vi "DB - T-SQL Query.vi"(8 "error in (no error)":errorcluster, 10 "T-SQL":string, 11 "connection reference":T1) -> (0 "error out":errorcluster, 2 "2D data":string[][](array[string]), 3 "connection reference":T1)   [LabVIEW 2020]
uses:
  <vilib>/addons/database/Connection.llb/Conn ObjectReference.ctl
  <vilib>/addons/database/Connection.llb/Conn Execute.vi
  <vilib>/addons/database/Recordset.llb/Rec Fetch Recordset Data (R).vi
  <vilib>/addons/database/Recordset.llb/Rec Destroy - Connection.vi
  <vilib>/addons/database/NI_Database_API.lvlib
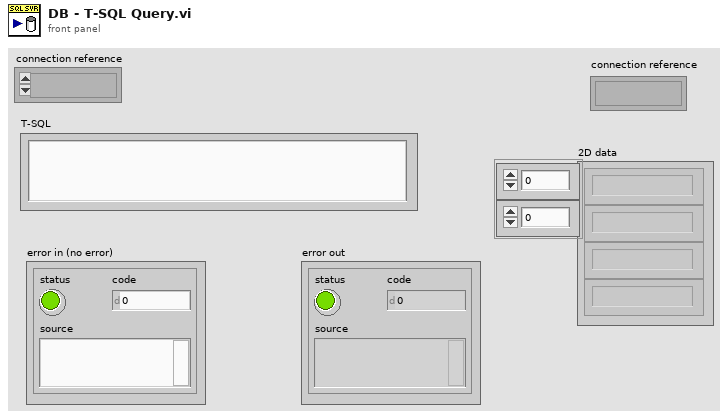
[diagram p1: front panel]
types:
  T1 = typedef "NI_Database_API.lvlib/Conn ObjectReference.ctl" = refnum<k1>
  T2 = typedef "NI_Database_API.lvlib/Rec ObjectReference.ctl" = refnum<k1>
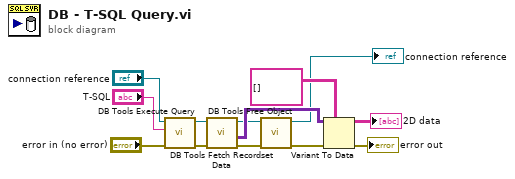
[diagram p0: block diagram]
diagram:
  n1 = call-poly <vilib>:"DB Tools Execute Query.vi"("error in (no error)"="error in (no error)", "SQL query"="T-SQL", "connection reference"="connection reference") -> ("error out"=w8:errorcluster, "recordset reference"=w7:T2)  [unwired: 5 in]
  n2 = call-poly <vilib>:"DB Tools Fetch Recordset Data.vi"("error in (no error)"=w8, "recordset reference"=w7) -> ("error out"=w6:errorcluster, "recordset data"=w12:variant[][], "recordset reference out"=w5:T2)  [unwired: 3 in]
  n3 = call-poly <vilib>:"DB Tools Free Object.vi"("error in (no error)"=w6, "recordset reference"=w5) -> ("error out"=w13:errorcluster, "connection reference"=→"connection reference":T1)  [unwired: 8 in]
  n4 = Variant To Data(error in=w13, type=string[][] [], Variant=w12) -> (data=→"2D data":string[][], error out=→"error out":errorcluster)
